vi "SortByIndex.vi"(4 "sortOrder":i32[](array[numeric]), 5 "1DstringIn":string[](array[string]), 6 "1Din":dbl[](array[numeric]), 8 "2Din":dbl[][](array[numeric])) -> (0 "1DstringOut":string[](array[string]), 1 "1Dout":dbl[](array[numeric]), 3 "2Dout":dbl[][](array[numeric]))   [LabVIEW 2021]
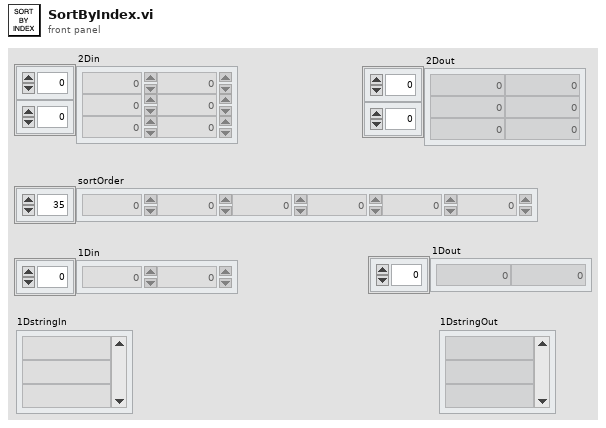
[diagram p1: front panel]
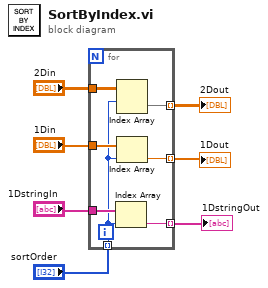
[diagram p0: block diagram]
diagram:
  n1 = for {
    tunnel: "2Din" -> [w14]
    tunnel: "sortOrder" -> [w8] mode=indexing
    tunnel: [w13] -> w7 mode=indexing
    tunnel: "1Din" -> [w12]
    tunnel: [w11] -> w3 mode=indexing
    tunnel: [w10] -> w2 mode=indexing
    tunnel: "1DstringIn" -> [w9]
    n2 = Index Array(array=w9, index=w8) -> (element=w10:string)
    n3 = Index Array(array=w14, index (row)=w8) -> (element=w13:dbl[])  [unwired: 1 in]
    n4 = Index Array(array=w12, index=w8) -> (element=w11:dbl)
  }
  "2Dout" <- w7
  "1Dout" <- w3
  "1DstringOut" <- w2
